vi "eventToClient.vi"(8 "error in (no error)":errorcluster, 10 "Event":T1, 11 "TcpServerCmd in":refnum<class "TcpServerCmd.lvclass">) -> (0 "error out":errorcluster, 3 "TcpServerCmd out":refnum<class "TcpServerCmd.lvclass">)   [LabVIEW 2018, in "TcpServerCmd.lvclass"]
doc: "Send an Event to the TCP Client."
uses:
  TcpServerCmd.lvclass
  home/pcortes/github/ts_labview_tcp_json/src/TcpServerBase/TcpServerBase.lvclass
  typedef/eventTypeDef.ctl
  TcpServerBase/typedef/tcpPacketTypeDef.ctl
  TcpServerBase/typedef/msgTypeEnum.ctl
  TcpServerBase/TcpServerBase.lvclass
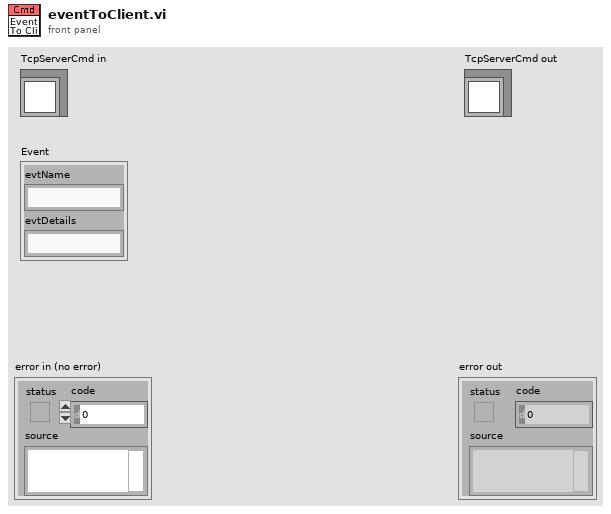
[diagram p1: front panel]
types:
  T1 = typedef "TcpServerCmd.lvclass/eventTypeDef.ctl" = cluster{"evtName":string, "evtDetails":string}
  T2 = typedef "TcpServerBase.lvclass/msgTypeEnum.ctl" = enum16{"event", "telemetry"}
  T3 = typedef "TcpServerBase.lvclass/tcpPacketTypeDef.ctl" = cluster{"packet":string, "firstPacket":bool, "firstConnection":bool}
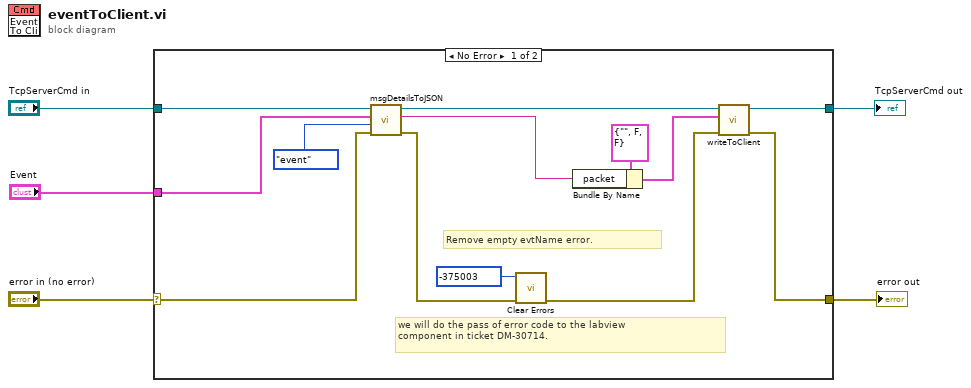
[diagram p0: block diagram]
diagram:
  n1 = case shown="No Error" "error in (no error)" {
    selector: "error in (no error)" -> [w12 w20]
    tunnel: [w17 w20] -> w4
    tunnel: [w18 w19] -> w2
    tunnel: "TcpServerCmd in" -> [w14 w19]
    tunnel: "Event" -> [w7 _]
    frame No Error {
      # "we will do the pass of error code to the labview \ncomponent in ticket DM-30714."
      # "Remove empty evtName error."
      n2 = call "msgDetailsToJSON.vi"("error in (no error)"=w12, "msgTypeEnum"=msgTypeEnum."event", "msgTypeDef"=w7, "TcpServerBase in"=w14) -> ("error out"=w10:errorcluster, "JSON string"=w9:string, "TcpServerBase out"=w13:refnum<class "TcpServerCmd.lvclass">)  [unwired: 5 in]
      n3 = call <vilib>:"Clear Errors.vi"("error in (no error)"=w10, "specific error code to clear (0: all)"=-375003) -> ("error out"=w8:errorcluster)  [unwired: 4 in, 1 out]
      n4 = Bundle By Name(cluster=T3 {"packet"="", "firstPacket"=FALSE, "firstConnection"=FALSE} ("packetConnID"), "packet"=w9) -> (w15:T3)
      n5 = call "writeToClient.vi"("error in (no error)"=w8, "tcpPacket"=w15, "tcpServerCmd in"=w13) -> ("error out"=w17:errorcluster, "tcpServerCmd out"=w18:refnum<class "TcpServerCmd.lvclass">)  [unwired: 7 in]
    }
    frame Error {
    }
  }
  "error out" <- w4
  "TcpServerCmd out" <- w2
